vi "Solution.vi"() -> ()   [LabVIEW 2020]
panel:
  out "result":i32
  in  "data?":bool
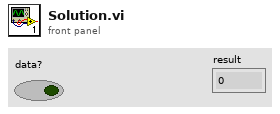
[diagram p1: front panel]
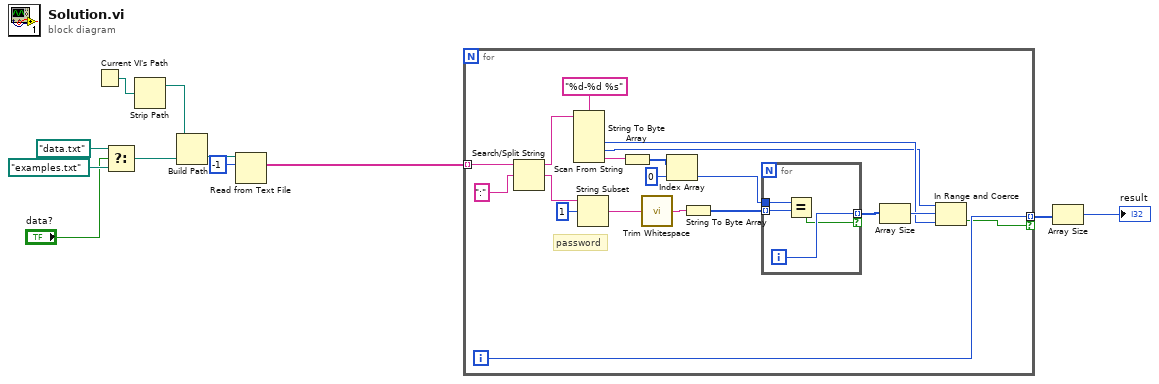
[diagram p0: block diagram]
diagram:
  n1 = Current VI's Path() -> (path=w7:path)
  n2 = Select(t=path "data.txt", s="data?", f=path "examples.txt") -> (s? t:f=w8:path)
  n3 = Strip Path(path=w7) -> (stripped path=w6:path)  [unwired: 1 out]
  n4 = Build Path(base path=w6, name or relative path=w8) -> (appended path=w5:path)
  n5 = Read from Text File(file (use dialog)=w5, count=-1) -> (text=w1:string[])  [unwired: 2 in, 3 out]
  n6 = for {
    tunnel: w1 -> [w30] mode=indexing
    tunnel: [w14] -> w4 mode=indexing if=w13
    i -> [w14]
    # "password"
    n7 = Search/Split String(string=w30, search string/char (-)=":") -> (substring before match=w25:string, match + rest of string=w28:string)  [unwired: 1 in, 1 out]
    n8 = Scan From String(format string="%d-%d %s", input string=w25) -> (output 1=w16:i32, output 2=w15:i32, output 3=w22:string)  [unwired: 5 in, 3 out]
    n9 = String Subset(string=w28, offset (0)=1) -> (substring=w24:string)  [unwired: 1 in]
    n10 = String To Byte Array(string=w22) -> (unsigned byte array=w21:u8[])
    n11 = call <vilib>:"Trim Whitespace.vi"("string"=w24) -> ("trimmed string"=w12:string)  [unwired: 1 in]
    n12 = Index Array(array=w21, index=0) -> (element=w19:u8)
    n13 = String To Byte Array(string=w12) -> (unsigned byte array=w23:u8[])
    n14 = for {
      tunnel: w23 -> [w34] mode=indexing
      tunnel: w19 -> [w33]
      tunnel: [w32] -> w18 mode=indexing if=w31
      i -> [w32]
      n15 = Equal?(x=w33, y=w34) -> (x = y?=w31:bool)
    }
    n16 = Array Size(array=w18) -> (size(s)=w17:i32)
    n17 = In Range and Coerce(upper limit=w15, x=w17, lower limit=w16) -> (In Range?=w13:bool)  [unwired: 1 out]
  }
  n18 = Array Size(array=w4) -> (size(s)=→"result":i32)
